vi "Create Clusters for Node Type Definitions.vi"(7 "Settings Cluster Path":path, 8 "error in":errorcluster, 11 "Nodes":refnum<k20>[](array[refnum])) -> (0 "error out":errorcluster, 1 "Node Types":string[](array[string]), 2 "Node Clusters":refnum<vi>[](array[refnum]), 3 "Nodes":refnum<k20>[](array[refnum]))   [LabVIEW 2026, in "XML Parser.lvlib"]
uses:
  XML Parser.lvlib
  <resource>/objmgr/DOMUserDefRef.rc
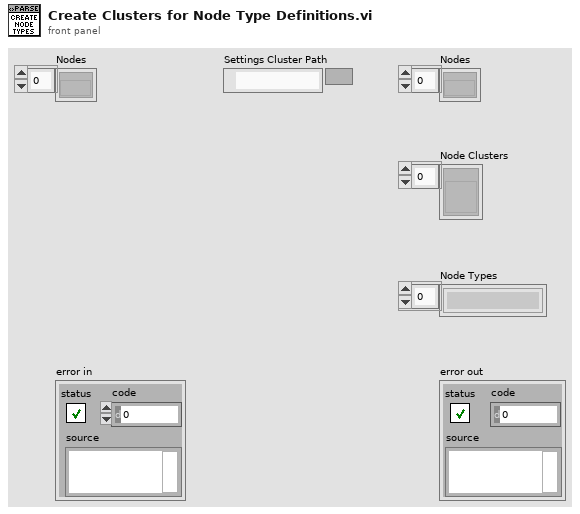
[diagram p1: front panel]
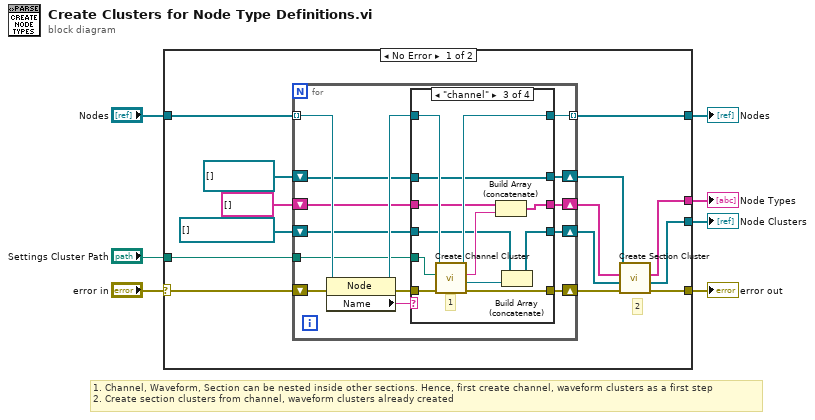
[diagram p0: block diagram]
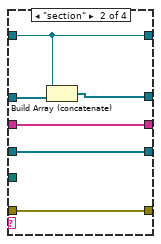
[diagram p3: hidden frame]
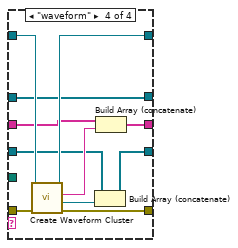
[diagram p4: hidden frame]
diagram:
  # "1. Channel, Waveform, Section can be nested inside other sections. Hence, first create channel, waveform clusters as a first step\n2. Create section clusters from channel, waveform clusters already created"
  n1 = case shown="No Error" "error in" {
    selector: "error in" -> [w21 w71]
    tunnel: [w19 w71] -> w7
    tunnel: [w18 w70] -> w5
    tunnel: "Nodes" -> [w17 w70]
    tunnel: [w10 _] -> w3
    tunnel: [w9 _] -> w2
    tunnel: "Settings Cluster Path" -> [w8 _]
    frame No Error {
      # "2"
      n2 = for {
        tunnel: [w30] -> w18 mode=indexing
        tunnel: w17 -> [w32] mode=indexing
        shift-right: [w34] -> w20
        shift-left: w21 -> [w35]
        shift-right: [w29] -> w13
        shift-left: refnum<k20>[] [] ("Sections") -> [w28]
        shift-right: [w27] -> w11
        shift-left: string[] [] ("Node Types") -> [w26]
        shift-right: [w25] -> w12
        shift-left: refnum<vi>[] [] ("Node Clusters") -> [w24]
        tunnel: w8 -> [w22]
        n3 = property class="Node"(reference=w32, error in=w35) -> (reference out=w31:refnum<k20>, error out=w33:errorcluster, "Name"=w23:string)
        n4 = case shown="\"channel\"" w23 {
          tunnel: w31 -> [w39 w43 w56 w67]
          tunnel: [w40 w46 w57 w68] -> w34
          tunnel: w33 -> [w40 w46 w58 w69]
          tunnel: [w39 w43 w55 w66] -> w30
          tunnel: [w38 w45 w54 w65] -> w29
          tunnel: w28 -> [w38 w44 w54 w65]
          tunnel: [w37 w42 w51 w62] -> w27
          tunnel: w26 -> [w37 w42 w52 w64]
          tunnel: [w36 w41 w49 w61] -> w25
          tunnel: w24 -> [w36 w41 w48 w59]
          tunnel: w22 -> [_ _ w47 _]
          frame Default {
          }
          frame "section" {
            n5 = Build Array (concatenate)(w43, w44) -> (w45:refnum<k20>[])
          }
          frame "channel" {
            # "1"
            n6 = call "Create Channel Cluster.vi"("error in"=w58, "Settings Cluster Path"=w47, "Node"=w56) -> ("error out"=w57:errorcluster, "Clust Refnum"=w50:refnum<vi>, "Channel Type"=w53:string, "Node"=w55:refnum<k20>)  [unwired: 5 in]
            n7 = Build Array (concatenate)(w52, w53) -> (w51:string[])
            n8 = Build Array (concatenate)(w48, w50) -> (w49:refnum<vi>[])
          }
          frame "waveform" {
            n9 = call "Create Waveform Cluster.vi"("error in"=w69, "Node"=w67) -> ("error out"=w68:errorcluster, "Clust Refnum"=w60:refnum<vi>, "Waveform Type"=w63:string, "Node"=w66:refnum<k20>)  [unwired: 6 in]
            n10 = Build Array (concatenate)(w59, w60) -> (w61:refnum<vi>[])
            n11 = Build Array (concatenate)(w64, w63) -> (w62:string[])
          }
        }
      }
      n12 = call "Create Section Cluster.vi"("error in"=w20, "Node Clusters"=w12, "Node Types"=w11, "Sections"=w13) -> ("error out"=w19:errorcluster, "Node Clusters"=w9:refnum<vi>[], "Node Types"=w10:string[])  [unwired: 4 in, 1 out]
    }
    frame Error {
    }
  }
  "error out" <- w7
  "Nodes" <- w5
  "Node Types" <- w3
  "Node Clusters" <- w2
